vi "Calculate Line Distance.vi"(9 "error in (no error)":errorcluster, 11 "Points":T1[](array[typedef])) -> (1 "error out":errorcluster, 2 "Distance":dbl, 3 "Points Out":T1[](array[typedef]))   [LabVIEW 2019, in "Tool Path.lvclass"]
uses:
  Tool Path.lvclass
  Parse/PathCommands/Point.ctl
  Parse/PathCommands/PathCommands.lvclass
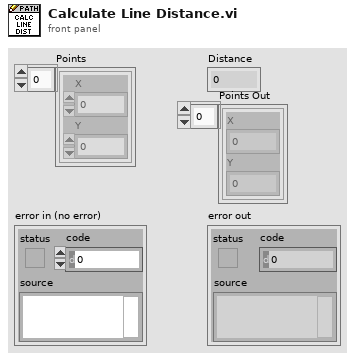
[diagram p1: front panel]
types:
  T1 = typedef "PathCommands.lvclass/Point.ctl" = cluster{"X":dbl, "Y":dbl}
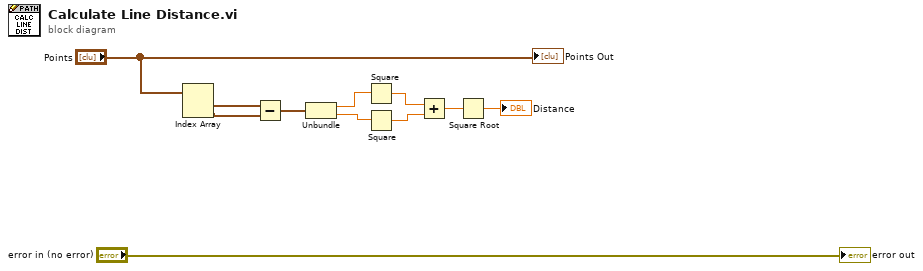
[diagram p0: block diagram]
diagram:
  n1 = Index Array(array="Points") -> (element #1=w9:T1, element #2=w8:T1)  [unwired: 2 in]
  n2 = Subtract(x=w9, y=w8) -> (x-y=w7:T1)
  n3 = Unbundle(w7) -> ("X"=w6:dbl, "Y"=w5:dbl)
  n4 = Square(x=w6) -> (x^2=w4:dbl)
  n5 = Square(x=w5) -> (x^2=w3:dbl)
  n6 = Add(x=w4, y=w3) -> (x+y=w2:dbl)
  n7 = Square Root(x=w2) -> (sqrt(x)=→"Distance":dbl)
  "error out" <- "error in (no error)"
  "Points Out" <- "Points"
